vi "db_transactions_update.vi"(0 "UDL PATH IN":path, 1 "TABLE NAME":string, 2 "VALUES":cluster{"FIELDS":string[], "VALUES":string[]}, 3 "CONDITION":cluster{"FIELD":string, "VALUE":string}, 4 "MODE":bool, 5 "ERROR IN":errorcluster) -> (14 "UDL PATH OUT":path, 19 "ERROR OUT":errorcluster)   [LabVIEW 2018, in "db_lib R3.lvlib"]
uses:
  db_lib R3.lvlib
  <vilib>/addons/database/Connection.llb/DB Tools Open Connec (Path).vi
  <vilib>/addons/database/Connection.llb/Conn Execute.vi
  <vilib>/addons/database/Recordset.llb/Rec Destroy - Connection.vi
  <vilib>/addons/database/NI_Database_API.lvlib
panel:
  # "UPDATE [table_name] SET [values] WHERE [condition];"
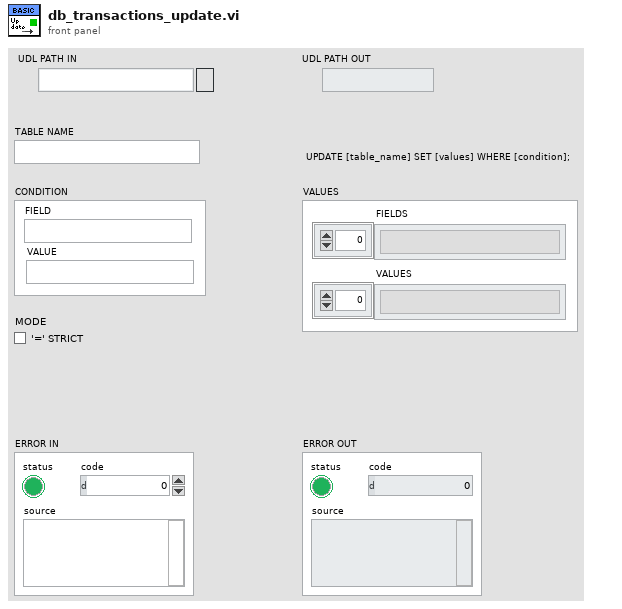
[diagram p1: front panel]
types:
  T1 = typedef "NI_Database_API.lvlib/Conn ObjectReference.ctl" = refnum<k1>
  T2 = typedef "NI_Database_API.lvlib/Rec ObjectReference.ctl" = refnum<k1>
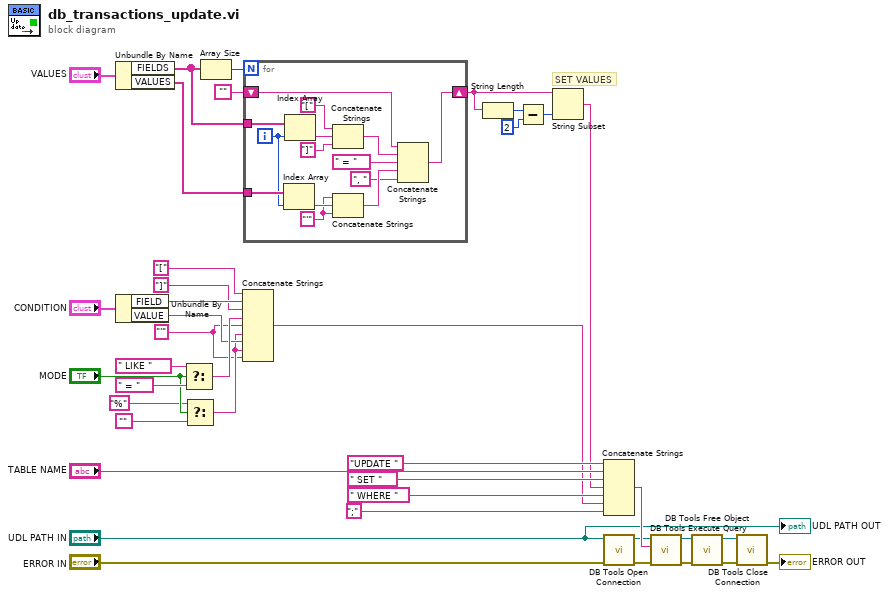
[diagram p0: block diagram]
diagram:
  w1 = "'" ("string")
  # "SET VALUES"
  n1 = Unbundle By Name("VALUES") -> ("FIELDS"=w32:string[], "VALUES"=w31:string[])
  n2 = Unbundle By Name("CONDITION") -> ("FIELD"=w25:string, "VALUE"=w3:string)
  n3 = Select(t=" LIKE ", s="MODE", f=" = ") -> (s? t:f=w23:string)
  n4 = Select(t="%", s="MODE", f="") -> (s? t:f=w2:string)
  n5 = Array Size(array=w32) -> (size(s)=w33:i32)
  n6 = Concatenate Strings("[" ("string"), w25, "]" ("string"), w23, w1, w2, w3, w2, w1) -> (w22:string)
  n7 = for {
    N: w33 -> [_]
    tunnel: w32 -> [w53]
    tunnel: w31 -> [w49]
    shift-right: [w41] -> w29
    shift-left: "" -> [w40]
    i -> [w48]
    w46 = "'" ("string")
    n8 = Index Array(array=w49, index=w48) -> (element=w47:string)
    n9 = Index Array(array=w53, index=w48) -> (element=w52:string)
    n10 = Concatenate Strings("[" ("string"), w52, "]" ("string")) -> (w45:string)
    n11 = Concatenate Strings(w46, w47, w46) -> (w43:string)
    n12 = Concatenate Strings(w40, w45, " = " ("string"), w43, ", " ("string")) -> (w41:string)
  }
  n13 = String Length(string=w29) -> (length=w11:i32)
  n14 = Subtract(x=w11, y=2) -> (x-y=w9:i32)
  n15 = String Subset(string=w29, length (rest)=w9) -> (substring=w28:string)  [unwired: 1 in]
  n16 = Concatenate Strings("UPDATE ", "TABLE NAME", " SET ", w28, " WHERE ", w22, ";" ("string")) -> (w36:string)
  n17 = call-poly <vilib>:"DB Tools Open Connection.vi"("error in (no error)"="ERROR IN", "connection information"="UDL PATH IN") -> ("error out"=w18:errorcluster, "connection reference"=w19:T1)  [unwired: 6 in]
  n18 = call-poly <vilib>:"DB Tools Execute Query.vi"("error in (no error)"=w18, "SQL query"=w36, "connection reference"=w19) -> ("error out"=w16:errorcluster, "recordset reference"=w17:T2)  [unwired: 5 in]
  n19 = call-poly <vilib>:"DB Tools Free Object.vi"("error in (no error)"=w16, "recordset reference"=w17) -> ("error out"=w15:errorcluster, "connection reference"=w14:T1)  [unwired: 8 in]
  n20 = call <vilib>:"DB Tools Close Connection.vi"("error in (no error)"=w15, "connection reference"=w14) -> ("error out"=→"ERROR OUT":errorcluster)  [unwired: 5 in]
  "UDL PATH OUT" <- "UDL PATH IN"
